vi "粘贴.vi"(8 "error in (no error)":errorcluster caption="错误输入（无错误）", 11 "程序 输入":refnum<class "程序.lvclass">) -> (0 "error out":errorcluster caption="错误输出", 3 "程序 输出":refnum<class "程序.lvclass">)   [LabVIEW 2018, in "程序.lvclass"]
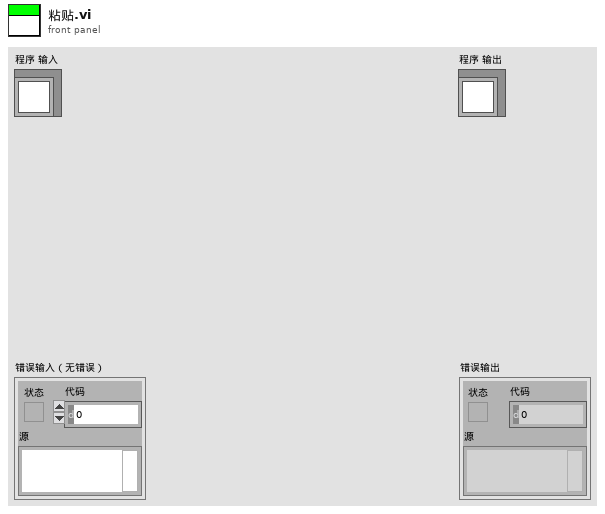
[diagram p1: front panel]
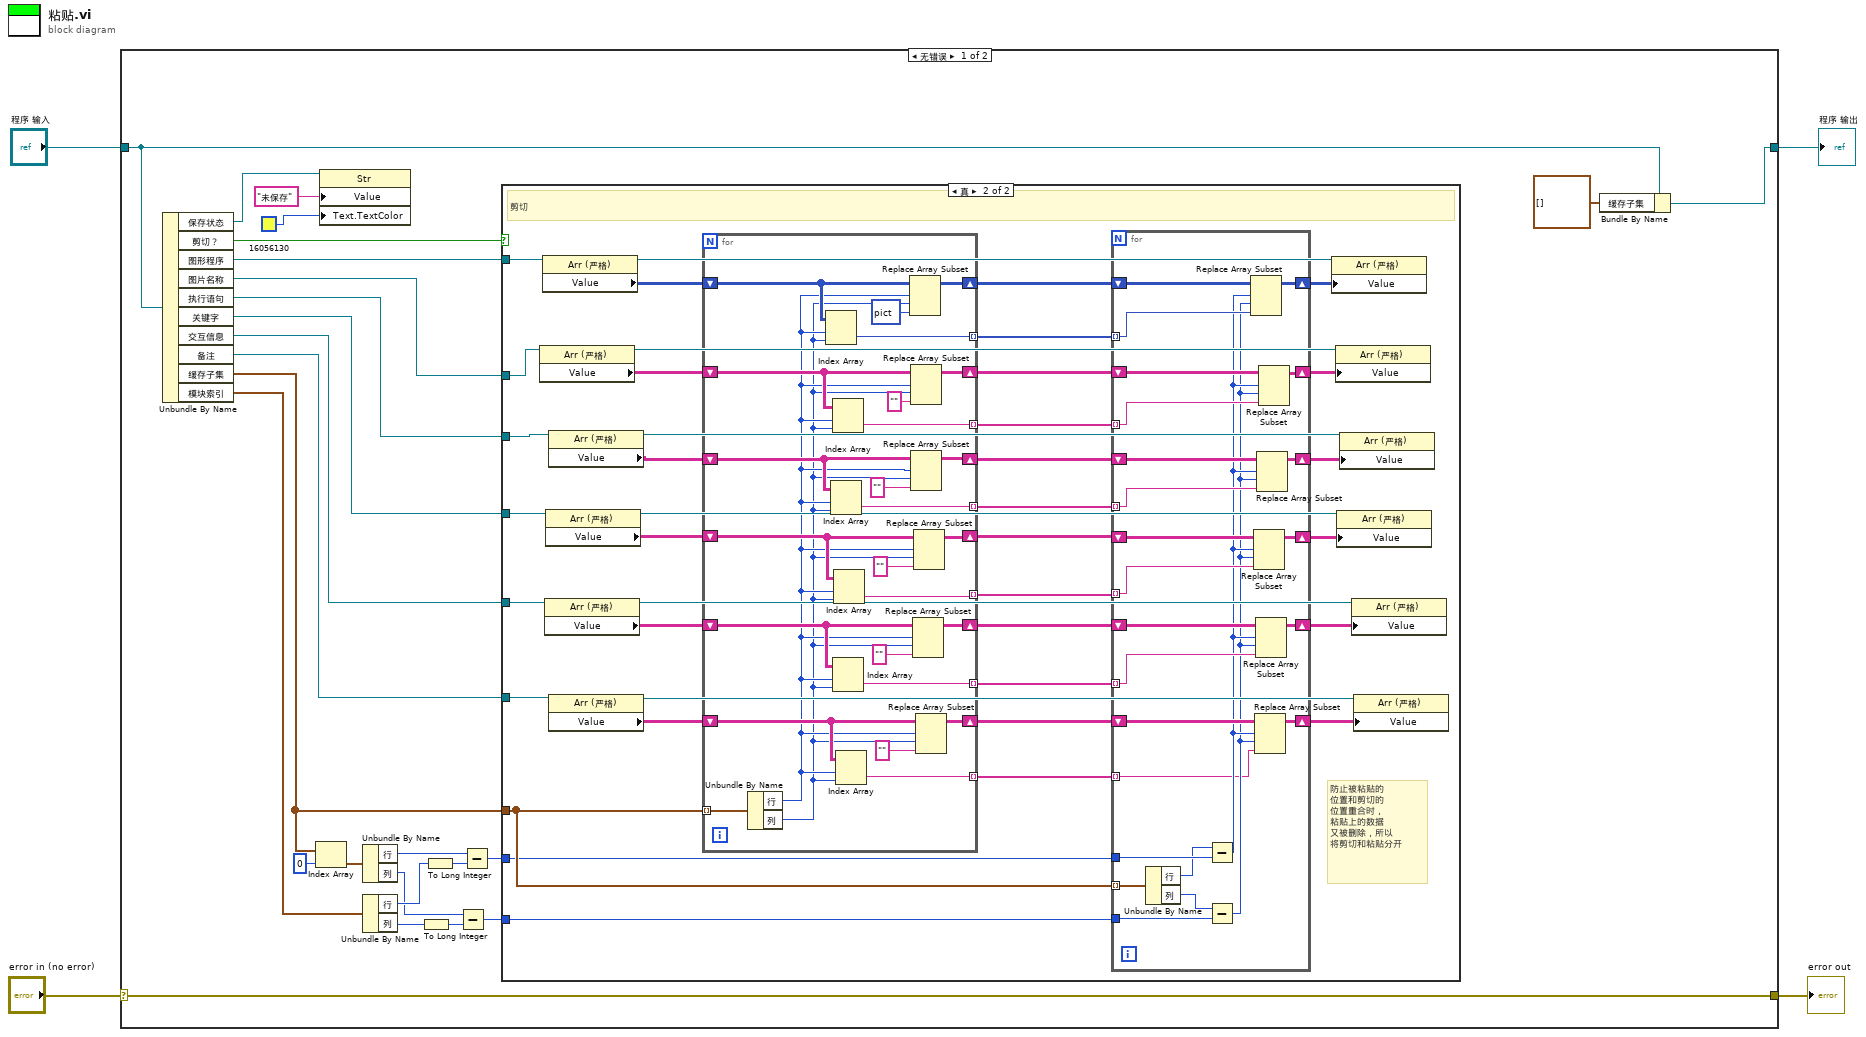
[diagram p0: block diagram]
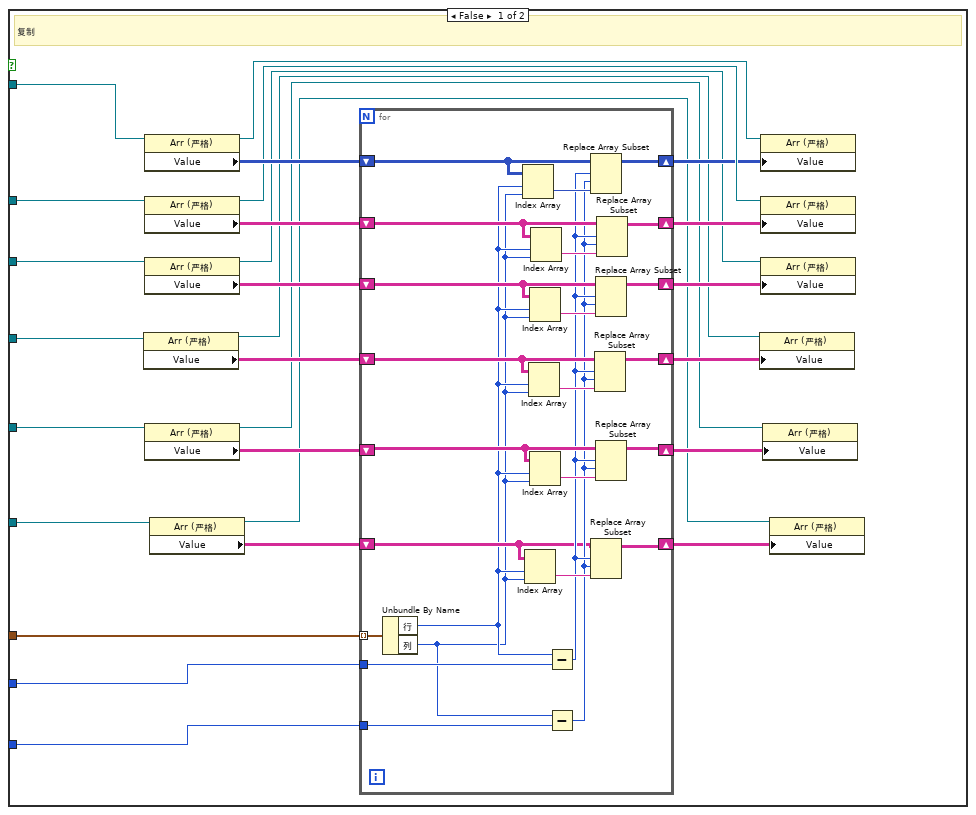
[diagram p2: hidden frame]
diagram:
  n1 = case shown="无错误" "error in (no error)" {
    selector: "error in (no error)" -> [w30 w175]
    tunnel: [w30 w175] -> w3
    tunnel: [w5 w174] -> w1
    tunnel: "程序 输入" -> [w7 w174]
    frame No Error {
      n2 = Unbundle By Name(w7) -> ("保存状态"=w8:refnum<vi>, "剪切？"=w19:bool, "图形程序"=w18:refnum<vi>, "图片名称"=w17:refnum<vi>, "执行语句"=w16:refnum<vi>, "关键字"=w13:refnum<vi>, "交互信息"=w12:refnum<vi>, "备注"=w11:refnum<vi>, "缓存子集"=w14:cluster{"行":i32, "列":i32}[], "模块索引"=w15:cluster{"列":u32, "行":u32})
      n3 = Index Array(array=w14, index=0 ("索引")) -> (element=w29:cluster{"行":i32, "列":i32})
      n4 = property class="Str"(reference=w8, "Value"="未保存" ("值"), "Text.TextColor"=u32 16056130) -> ()  [unwired: 1 in, 2 out]
      n5 = Unbundle By Name(w29) -> ("行"=w28:i32, "列"=w24:i32)
      n6 = Unbundle By Name(w15) -> ("行"=w27:u32, "列"=w23:u32)
      n7 = To Long Integer(number=w23) -> (32bit integer=w25:i32)
      n8 = To Long Integer(number=w27) -> (32bit integer=w26:i32)
      n9 = Subtract(x=w24, y=w25) -> (x-y=w21:i32)
      n10 = Subtract(x=w28, y=w26) -> (x-y=w22:i32)
      n11 = case shown="真" w19 {
        tunnel: w18 -> [w54 w114]
        tunnel: w17 -> [w52 w112]
        tunnel: w16 -> [w50 w109]
        tunnel: w14 -> [w55 w121]
        tunnel: w22 -> [w57 w117]
        tunnel: w21 -> [w56 w116]
        tunnel: w13 -> [w40 w99]
        tunnel: w12 -> [w38 w94]
        tunnel: w11 -> [w34 w88]
        frame False {
          # "复制"
          n12 = property class="Arr (严格)"(reference=w40) -> (reference out=w39:refnum<vi>, "Value"=w41:string[][])  [unwired: 1 in, 1 out]
          n13 = property class="Arr (严格)"(reference=w54) -> (reference out=w48:refnum<vi>, "Value"=w53:picture[][])  [unwired: 1 in, 1 out]
          n14 = property class="Arr (严格)"(reference=w52) -> (reference out=w45:refnum<vi>, "Value"=w51:string[][])  [unwired: 1 in, 1 out]
          n15 = property class="Arr (严格)"(reference=w50) -> (reference out=w43:refnum<vi>, "Value"=w49:string[][])  [unwired: 1 in, 1 out]
          n16 = property class="Arr (严格)"(reference=w38) -> (reference out=w36:refnum<vi>, "Value"=w37:string[][])  [unwired: 1 in, 1 out]
          n17 = property class="Arr (严格)"(reference=w34) -> (reference out=w31:refnum<vi>, "Value"=w33:string[][])  [unwired: 1 in, 1 out]
          n18 = for {
            tunnel: w55 -> [w82] mode=indexing
            tunnel: w57 -> [w81]
            tunnel: w56 -> [w80]
            shift-right: [w75] -> w44
            shift-left: w53 -> [w76]
            shift-right: [w73] -> w47
            shift-left: w51 -> [w74]
            shift-right: [w71] -> w46
            shift-left: w49 -> [w72]
            shift-right: [w70] -> w42
            shift-left: w41 -> [w69]
            shift-right: [w66] -> w35
            shift-left: w37 -> [w65]
            shift-right: [w63] -> w32
            shift-left: w33 -> [w60]
            n19 = Unbundle By Name(w82) -> ("行"=w59:i32, "列"=w58:i32)
            n20 = Index Array(array=w76, index (row)=w59, index (col)=w58) -> (element=w79:picture)
            n21 = Index Array(array=w60, index (row)=w59, index (col)=w58) -> (element=w64:string)
            n22 = Index Array(array=w69, index (row)=w59, index (col)=w58) -> (element=w68:string)
            n23 = Index Array(array=w72, index (row)=w59, index (col)=w58) -> (element=w77:string)
            n24 = Index Array(array=w65, index (row)=w59, index (col)=w58) -> (element=w67:string)
            n25 = Index Array(array=w74, index (row)=w59, index (col)=w58) -> (element=w78:string)
            n26 = Subtract(x=w59, y=w81) -> (x-y=w62:i32)
            n27 = Subtract(x=w58, y=w80) -> (x-y=w61:i32)
            n28 = Replace Array Subset(array=w76, new element=w79, index (row)=w62, index (col)=w61) -> (w75:picture[][])
            n29 = Replace Array Subset(array=w60, new element=w64, index (row)=w62, index (col)=w61) -> (w63:string[][])
            n30 = Replace Array Subset(array=w69, new element=w68, index (row)=w62, index (col)=w61) -> (w70:string[][])
            n31 = Replace Array Subset(array=w72, new element=w77, index (row)=w62, index (col)=w61) -> (w71:string[][])
            n32 = Replace Array Subset(array=w65, new element=w67, index (row)=w62, index (col)=w61) -> (w66:string[][])
            n33 = Replace Array Subset(array=w74, new element=w78, index (row)=w62, index (col)=w61) -> (w73:string[][])
          }
          n34 = property class="Arr (严格)"(reference=w39, "Value"=w42) -> ()  [unwired: 1 in, 2 out]
          n35 = property class="Arr (严格)"(reference=w48, "Value"=w44) -> ()  [unwired: 1 in, 2 out]
          n36 = property class="Arr (严格)"(reference=w45, "Value"=w47) -> ()  [unwired: 1 in, 2 out]
          n37 = property class="Arr (严格)"(reference=w43, "Value"=w46) -> ()  [unwired: 1 in, 2 out]
          n38 = property class="Arr (严格)"(reference=w36, "Value"=w35) -> ()  [unwired: 1 in, 2 out]
          n39 = property class="Arr (严格)"(reference=w31, "Value"=w32) -> ()  [unwired: 1 in, 2 out]
        }
        frame True {
          # "防止被粘贴的\n位置和剪切的\n位置重合时，\n粘贴上的数据\n又被删除，所以\n将剪切和粘贴分开"
          # "剪切"
          n40 = property class="Arr (严格)"(reference=w112) -> (reference out=w102:refnum<vi>, "Value"=w111:string[][])  [unwired: 1 in, 1 out]
          n41 = property class="Arr (严格)"(reference=w114) -> (reference out=w103:refnum<vi>, "Value"=w113:picture[][])  [unwired: 1 in, 1 out]
          n42 = property class="Arr (严格)"(reference=w94) -> (reference out=w92:refnum<vi>, "Value"=w93:string[][])  [unwired: 1 in, 1 out]
          n43 = property class="Arr (严格)"(reference=w99) -> (reference out=w95:refnum<vi>, "Value"=w100:string[][])  [unwired: 1 in, 1 out]
          n44 = property class="Arr (严格)"(reference=w109) -> (reference out=w101:refnum<vi>, "Value"=w108:string[][])  [unwired: 1 in, 1 out]
          n45 = property class="Arr (严格)"(reference=w88) -> (reference out=w83:refnum<vi>, "Value"=w87:string[][])  [unwired: 1 in, 1 out]
          n46 = for {
            tunnel: w121 -> [w173] mode=indexing
            tunnel: [w170] -> w119 mode=indexing
            tunnel: [w169] -> w118 mode=indexing
            tunnel: [w168] -> w120 mode=indexing
            shift-right: [w167] -> w115
            shift-left: w113 -> [w166]
            shift-right: [w164] -> w110
            shift-left: w111 -> [w165]
            shift-right: [w162] -> w107
            shift-left: w108 -> [w163]
            tunnel: [w160] -> w96 mode=indexing
            shift-right: [w159] -> w97
            shift-left: w100 -> [w161]
            shift-right: [w155] -> w91
            shift-left: w93 -> [w154]
            tunnel: [w153] -> w90 mode=indexing
            shift-right: [w151] -> w85
            shift-left: w87 -> [w150]
            tunnel: [w147] -> w86 mode=indexing
            n47 = Unbundle By Name(w173) -> ("行"=w149:i32, "列"=w148:i32)
            n48 = Index Array(array=w166, index (row)=w149, index (col)=w148) -> (element=w169:picture)
            n49 = Index Array(array=w163, index (row)=w149, index (col)=w148) -> (element=w168:string)
            n50 = Index Array(array=w165, index (row)=w149, index (col)=w148) -> (element=w170:string)
            n51 = Index Array(array=w154, index (row)=w149, index (col)=w148) -> (element=w153:string)
            n52 = Index Array(array=w161, index (row)=w149, index (col)=w148) -> (element=w160:string)
            n53 = Index Array(array=w150, index (row)=w149, index (col)=w148) -> (element=w147:string)
            n54 = Replace Array Subset(array=w166, new element=picture data[5B] ("新元素/子数组"), index (row)=w149, index (col)=w148) -> (w167:picture[][])
            n55 = Replace Array Subset(array=w165, new element="" ("新元素/子数组"), index (row)=w149, index (col)=w148) -> (w164:string[][])
            n56 = Replace Array Subset(array=w163, new element="" ("新元素/子数组"), index (row)=w149, index (col)=w148) -> (w162:string[][])
            n57 = Replace Array Subset(array=w154, new element="" ("新元素/子数组"), index (row)=w149, index (col)=w148) -> (w155:string[][])
            n58 = Replace Array Subset(array=w161, new element="" ("新元素/子数组"), index (row)=w149, index (col)=w148) -> (w159:string[][])
            n59 = Replace Array Subset(array=w150, new element="" ("新元素/子数组"), index (row)=w149, index (col)=w148) -> (w151:string[][])
          }
          n60 = for {
            tunnel: w121 -> [w146] mode=indexing
            tunnel: w117 -> [w145]
            tunnel: w116 -> [w144]
            tunnel: w120 -> [w139] mode=indexing
            tunnel: w119 -> [w140] mode=indexing
            tunnel: w118 -> [w141] mode=indexing
            shift-right: [w137] -> w104
            shift-left: w115 -> [w138]
            shift-right: [w135] -> w105
            shift-left: w110 -> [w136]
            shift-right: [w133] -> w106
            shift-left: w107 -> [w134]
            tunnel: w96 -> [w130] mode=indexing
            shift-right: [w132] -> w98
            shift-left: w97 -> [w131]
            tunnel: w90 -> [w127] mode=indexing
            shift-right: [w128] -> w89
            shift-left: w91 -> [w129]
            tunnel: w86 -> [w122] mode=indexing
            shift-right: [w125] -> w84
            shift-left: w85 -> [w126]
            n61 = Unbundle By Name(w146) -> ("行"=w143:i32, "列"=w142:i32)
            n62 = Subtract(x=w143, y=w145) -> (x-y=w124:i32)
            n63 = Subtract(x=w142, y=w144) -> (x-y=w123:i32)
            n64 = Replace Array Subset(array=w138, new element=w141, index (row)=w124, index (col)=w123) -> (w137:picture[][])
            n65 = Replace Array Subset(array=w131, new element=w130, index (row)=w124, index (col)=w123) -> (w132:string[][])
            n66 = Replace Array Subset(array=w126, new element=w122, index (row)=w124, index (col)=w123) -> (w125:string[][])
            n67 = Replace Array Subset(array=w129, new element=w127, index (row)=w124, index (col)=w123) -> (w128:string[][])
            n68 = Replace Array Subset(array=w134, new element=w139, index (row)=w124, index (col)=w123) -> (w133:string[][])
            n69 = Replace Array Subset(array=w136, new element=w140, index (row)=w124, index (col)=w123) -> (w135:string[][])
          }
          n70 = property class="Arr (严格)"(reference=w103, "Value"=w104) -> ()  [unwired: 1 in, 2 out]
          n71 = property class="Arr (严格)"(reference=w102, "Value"=w105) -> ()  [unwired: 1 in, 2 out]
          n72 = property class="Arr (严格)"(reference=w95, "Value"=w98) -> ()  [unwired: 1 in, 2 out]
          n73 = property class="Arr (严格)"(reference=w101, "Value"=w106) -> ()  [unwired: 1 in, 2 out]
          n74 = property class="Arr (严格)"(reference=w92, "Value"=w89) -> ()  [unwired: 1 in, 2 out]
          n75 = property class="Arr (严格)"(reference=w83, "Value"=w84) -> ()  [unwired: 1 in, 2 out]
        }
      }
      n76 = Bundle By Name(cluster=w7, "缓存子集"=cluster{"行":i32, "列":i32}[] []) -> (w5:refnum<class "程序.lvclass">)
    }
    frame Error {
    }
  }
  "error out" <- w3
  "程序 输出" <- w1
